vi "data insert table.vi"(8 "error in (no error)":errorcluster, 10 "EXO message":T1, 11 "table":string="EXO") -> (0 "error out":errorcluster)   [LabVIEW 2016, in "EXO2-Sonde.lvlib"]
uses:
  EXO2-Sonde.lvlib
  <vilib>/addons/database/Auxilliary.llb/DB Tools Column Info.ctl
  <vilib>/addons/database/Auxilliary.llb/DB Tools DataTypes.ctl
  <vilib>/addons/database/NI_Database_API.lvlib
  <vilib>/Utility/VariantDataType/VariantType.lvlib
panel:
  in  "data in":T2
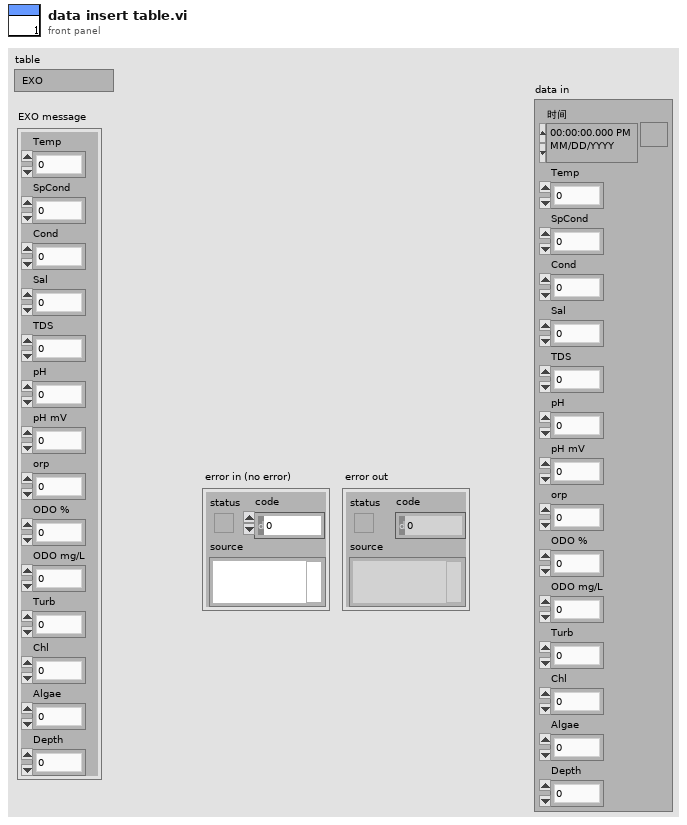
[diagram p1: front panel]
types:
  T1 = cluster{"Temp":dbl, "SpCond":dbl, "Cond":dbl, "Sal":dbl, "TDS":dbl, "pH":dbl, "pH mV":dbl, "orp":dbl, "ODO %":dbl, "ODO mg/L":dbl, "Turb":dbl, "Chl":dbl, "Algae":dbl, "Depth":dbl}
  T2 = cluster{"时间":timestamp, "Temp":dbl, "SpCond":dbl, "Cond":dbl, "Sal":dbl, "TDS":dbl, "pH":dbl, "pH mV":dbl, "orp":dbl, "ODO %":dbl, "ODO mg/L":dbl, "Turb":dbl, "Chl":dbl, "Algae":dbl, "Depth":dbl}
  T3 = typedef "NI_Database_API.lvlib/DB Tools Column Info.ctl" = cluster{"column name":string, "data type":T4, "size":i32, "allow null?":bool}
  T4 = typedef "NI_Database_API.lvlib/DB Tools DataTypes.ctl" = enum16{"String", "Long (I32)", "Single (SGL)", "Double (DBL)", "Date/Time", "Binary"}
  T5 = typedef "VariantType.lvlib/Type.ctl" = enum8{"Invalid Type", "Void", "I8", "I16", "I32", "I64", "U8", "U16", "U32", "U64", "Single Float", "Double Float", "Extended Float", "Single Complex", "Double Complex", "Extended Complex", "Enum U8", "Enum U16", "Enum U32", "Enum U64", "Single Float With Unit", "Double Float With Unit", "Extended Float With Unit", "Single Complex with Unit", "Double Complex with Unit", "Extended Complex with Unit", "Boolean", "String", "Path", "Picture", "Tag", "Array", "Cluster", "Variant", "LV Variant", "Waveform", "Timestamp", "Digital Waveform", "Digital Data", "ExpressData", "Refnum", "External Data", "VI", "Poly VI", "LabVIEW Class Instance", "Fixed Point"}
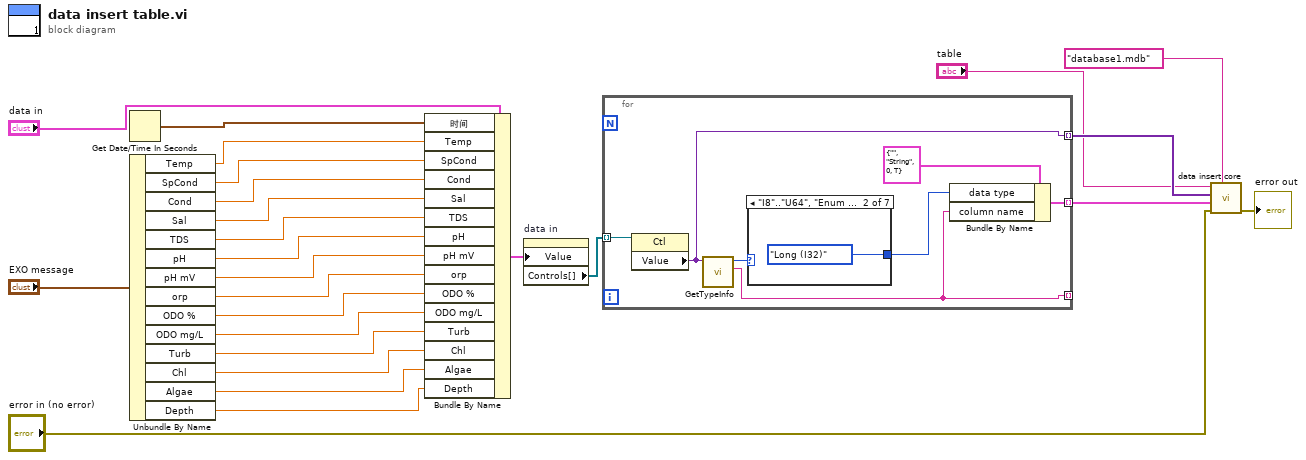
[diagram p0: block diagram]
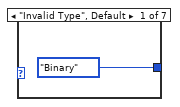
[diagram p2: hidden frame]
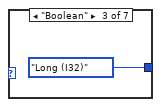
[diagram p3: hidden frame]
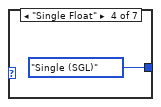
[diagram p4: hidden frame]
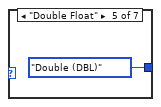
[diagram p5: hidden frame]
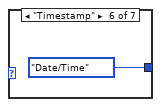
[diagram p6: hidden frame]
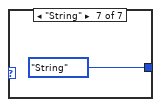
[diagram p7: hidden frame]
diagram:
  n1 = Get Date/Time In Seconds() -> (seconds since 1Jan1904=w2:timestamp)
  n2 = Unbundle By Name("EXO message") -> ("Temp"=w3:dbl, "SpCond"=w4:dbl, "Cond"=w5:dbl, "Sal"=w6:dbl, "TDS"=w7:dbl, "pH"=w8:dbl, "pH mV"=w9:dbl, "orp"=w10:dbl, "ODO %"=w11:dbl, "ODO mg/L"=w12:dbl, "Turb"=w13:dbl, "Chl"=w14:dbl, "Algae"=w15:dbl, "Depth"=w16:dbl)
  n3 = Bundle By Name(cluster="data in", "时间"=w2, "Temp"=w3, "SpCond"=w4, "Cond"=w5, "Sal"=w6, "TDS"=w7, "pH"=w8, "pH mV"=w9, "orp"=w10, "ODO %"=w11, "ODO mg/L"=w12, "Turb"=w13, "Chl"=w14, "Algae"=w15, "Depth"=w16) -> (w18:T2)
  n4 = property on="data in" class="Clust (严格)"("Value"=w18) -> ("Controls[]"=w22:refnum<vi>[])  [unwired: 2 in, 2 out]
  n5 = for {
    tunnel: w22 -> [w32] mode=indexing
    tunnel: [w27] -> w21 mode=indexing
    tunnel: [w28] -> w20 mode=indexing
    tunnel: [w26] -> _ mode=indexing
    n6 = property class="Ctl"(reference=w32) -> ("Value"=w27:variant)  [unwired: 1 in, 2 out]
    n7 = call <vilib>:"GetTypeInfo.vi"("Variant"=w27) -> ("Name"=w26:string, "Type Enum"=w30:T5)  [unwired: 6 in, 3 out]
    n8 = case shown="\"I8\"..\"U64\", \"Enum U8\"..\"Enum U64\"" w30 {
      tunnel: [DB_Tools_DataTypes."Binary" ("data type") DB_Tools_DataTypes."Long (I32)" ("data type") DB_Tools_DataTypes."Long (I32)" ("data type") DB_Tools_DataTypes."Single (SGL)" ("data type") DB_Tools_DataTypes."Double (DBL)" ("data type") DB_Tools_DataTypes."Date/Time" ("data type") DB_Tools_DataTypes."String" ("data type")] -> w29
      frame "Invalid Type", Default {
      }
      frame "I8".."U64", "Enum U8".."Enum U64" {
      }
      frame "Boolean" {
      }
      frame "Single Float" {
      }
      frame "Double Float" {
      }
      frame "Timestamp" {
      }
      frame "String" {
      }
    }
    n9 = Bundle By Name(cluster=T3 {"column name"="", "data type"=enum."String", "size"=0, "allow null?"=TRUE} ("column information"), "data type"=w29, "column name"=w26) -> (w28:T3)
  }
  n10 = call "data insert core.vi"("database"="database1.mdb", "error in (no error)"="error in (no error)", "column information"=w20, "data"=w21, "table"="table") -> ("error out"=→"error out":errorcluster)  [unwired: 6 in]
